vi "UPS_Monitor.vi"() -> ()   [LabVIEW 2023]
uses:
  Controls/Acquired_Datactl.ctl
  Controls/Queue_Operation_Select.ctl
  Controls/Acquired_Data.ctl
  Controls/State_and_Data.ctl
  Controls/File_Operation_Select.ctl
panel:
  out "Error_Out":errorcluster
  in  "Error_In":errorcluster
  in  "Tab Control":enum32{"PARAMETER", "DETAILS"}(tab)
  out "ACQUIRED_DATA":T1 {"Power_Consumption" scale=0.0..10.0; "Battery_Power" scale=0.0..10.0}
  out "Low_Power_Indicator":bool caption="Low Power Indicator"
  out "Waveform Graph":dbl[][](graph)
  in  "Record":bool
  in  "Stop":bool
  in  "Pause":bool
  in  "Start":bool
  # "UPS Monitor"
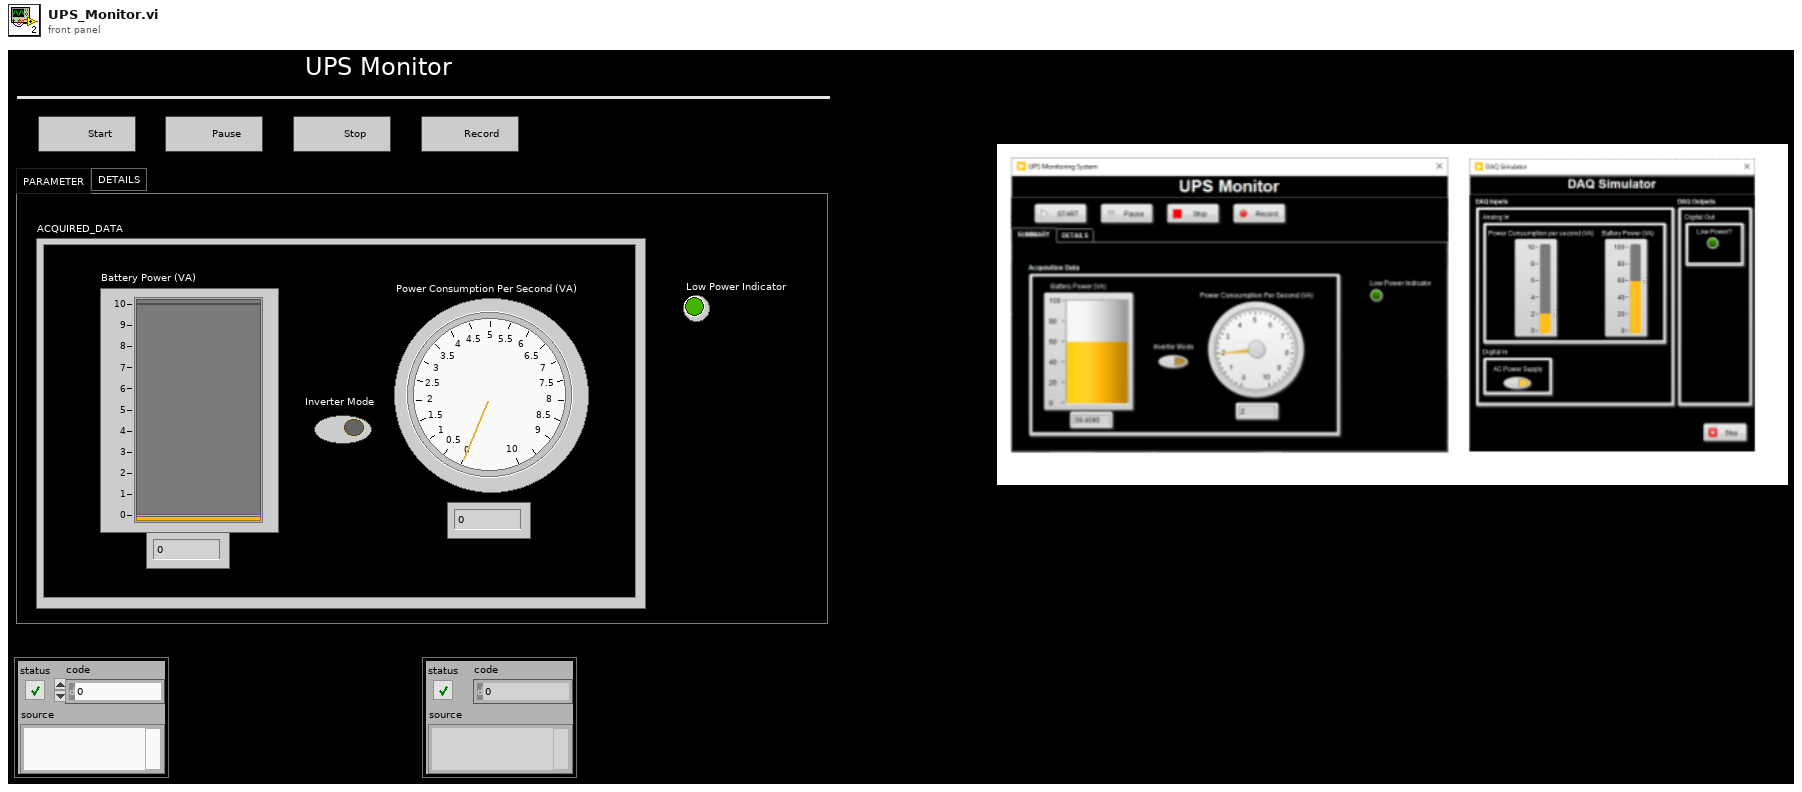
[diagram p1: front panel]
types:
  T1 = typedef "Acquired_Datactl.ctl" = cluster{"Battery_Power":dbl, "Power_Consumption":dbl, "Inverter_Mode":bool}
  T2 = typedef "Acquired_Data.ctl" = cluster{"Battery_Power":dbl, "Power_Consumption":dbl, "Inverter_Mode":bool}
  T3 = typedef "State_and_Data.ctl" = cluster{"State":string, "Data":variant}
  T4 = cluster{"ACQUIRED_DATA":T2, "Start":bool, "Pause":bool, "Record":bool, "Low_Power":bool, "Power_and_Power_Consumed":dbl[][], "State_and_Data_In":T3}
  T5 = typedef "Queue_Operation_Select.ctl" = enum16{"Obtain_Queue", "Enqueue", "Enqueue_First", "Enqueue_N", "Lossy_Enqueue", "Preview", "Queue_Status", "Dequeue", "Flush", "Release_Queue"}
  T6 = typedef "File_Operation_Select.ctl" = enum16{"Open", "Write", "Read", "Close"}
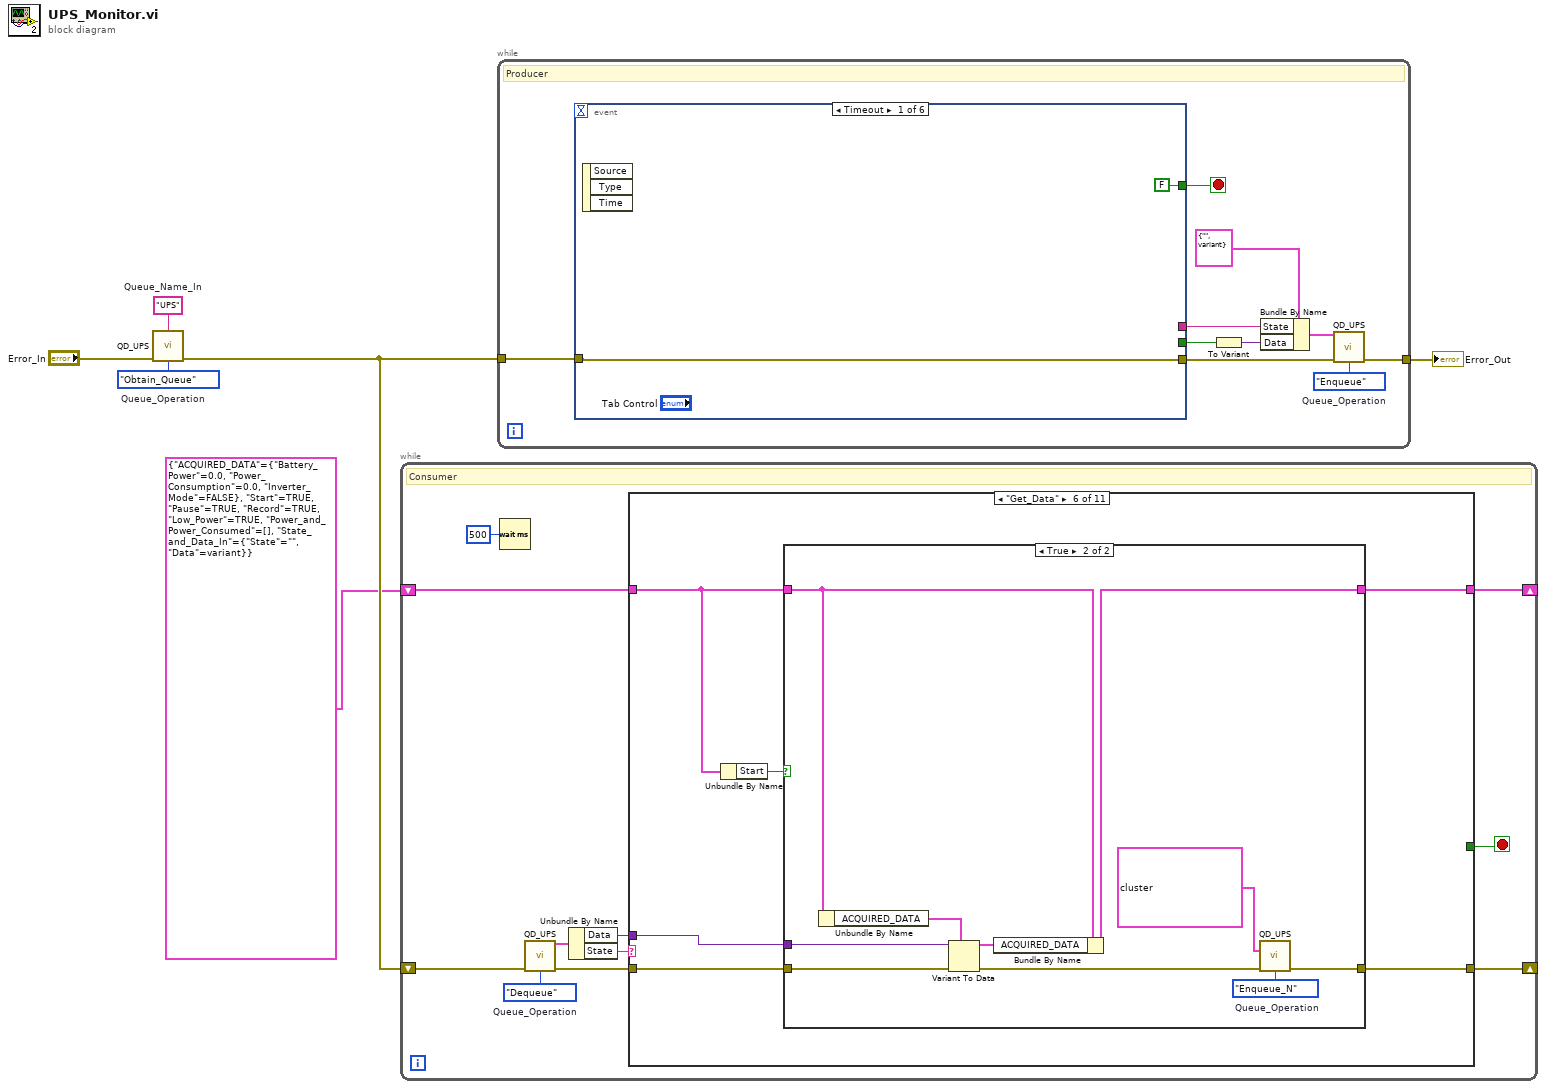
[diagram p0: block diagram]
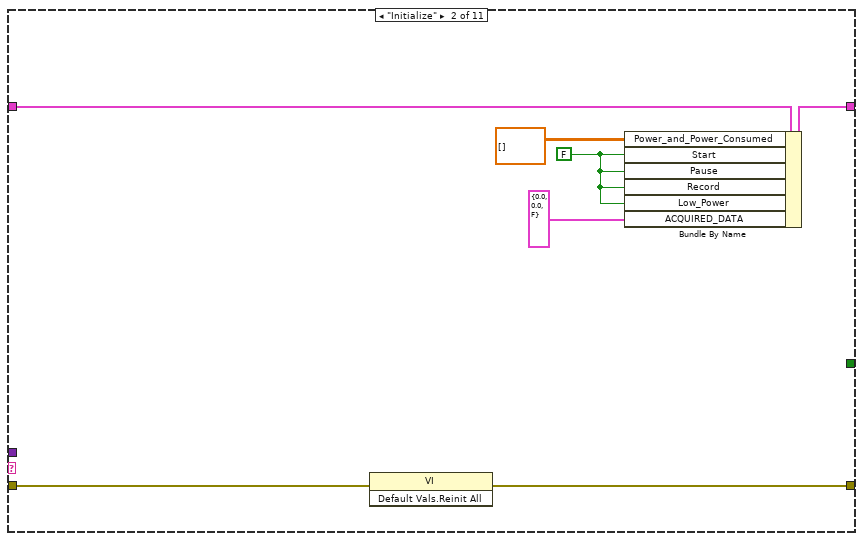
[diagram p3: hidden frame]
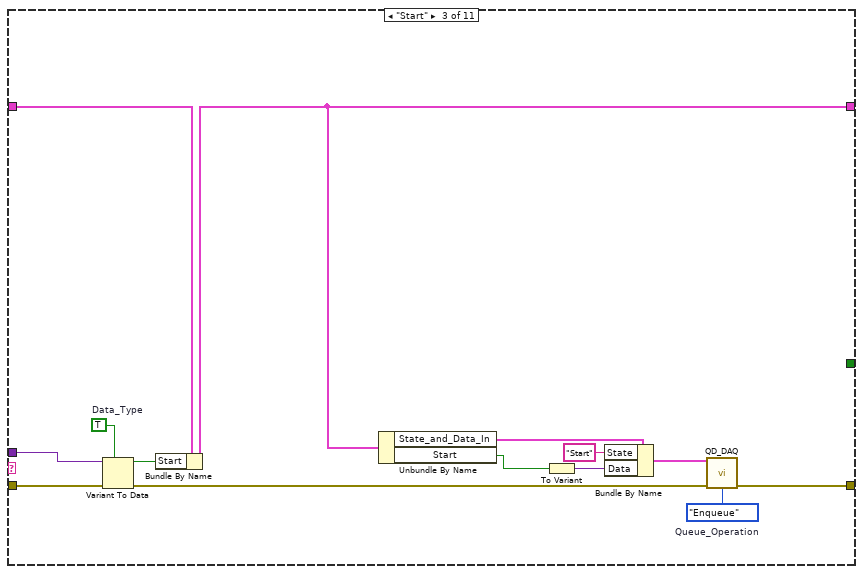
[diagram p4: hidden frame]
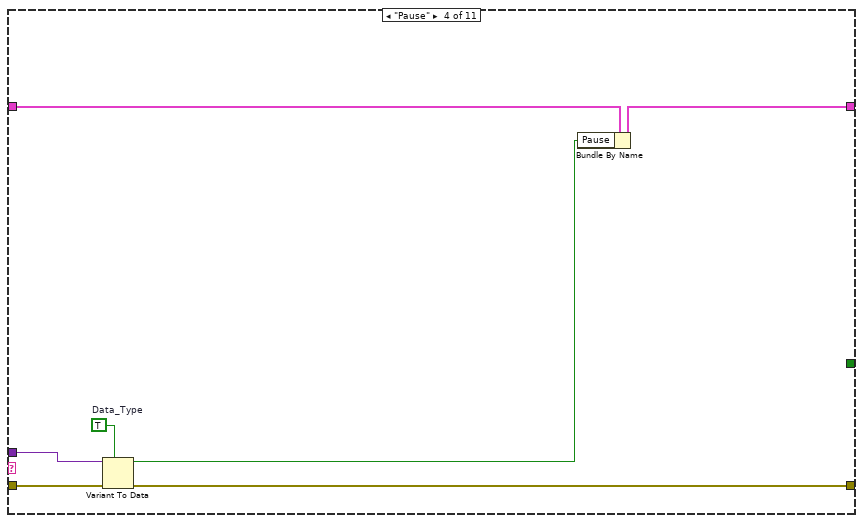
[diagram p5: hidden frame]
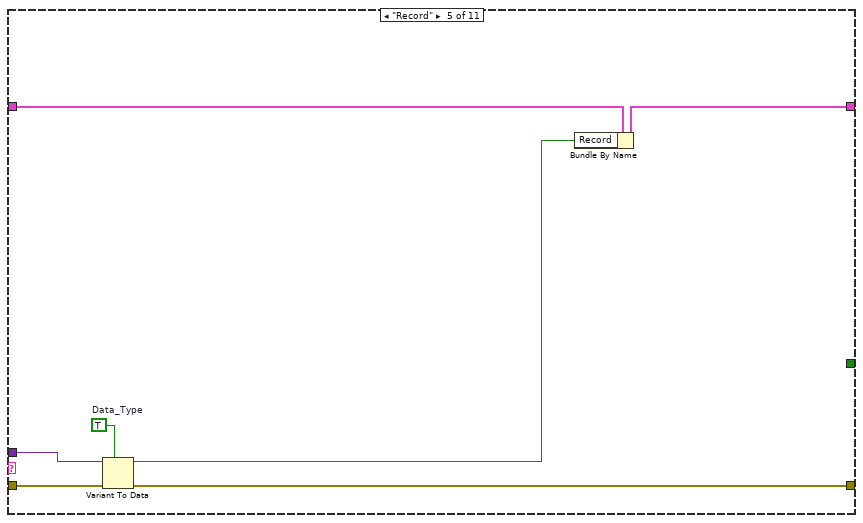
[diagram p6: hidden frame]
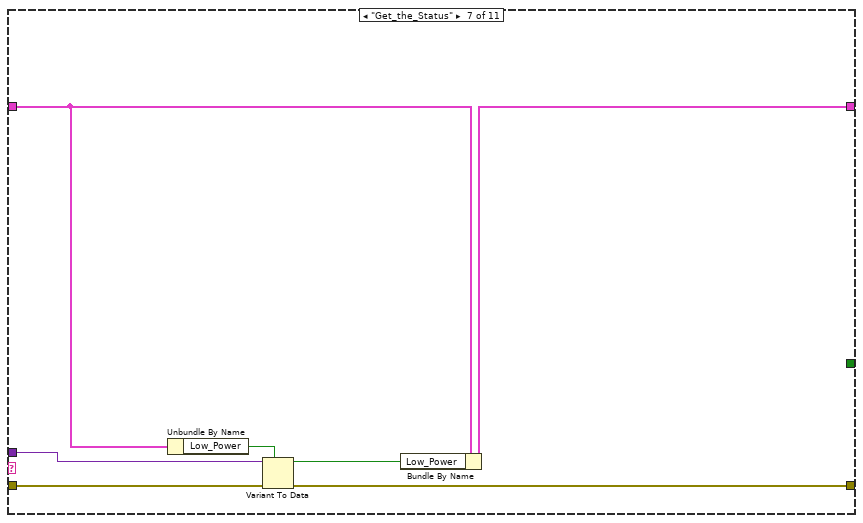
[diagram p8: hidden frame]
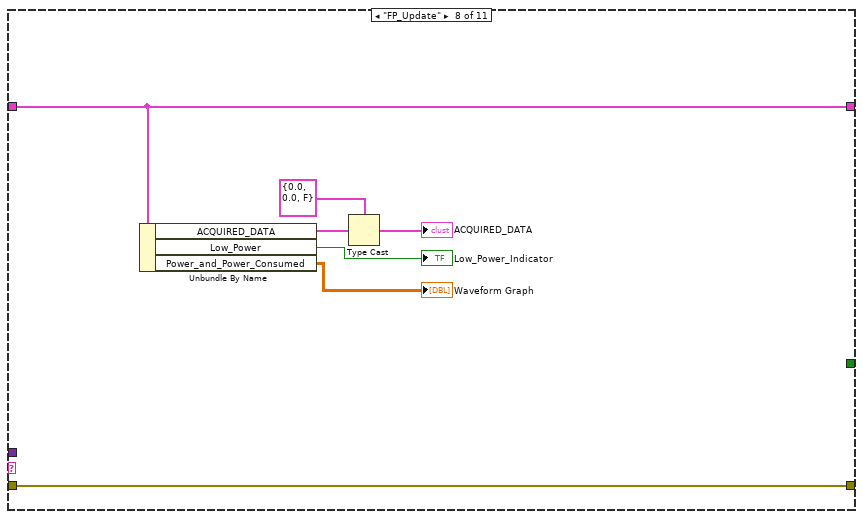
[diagram p9: hidden frame]
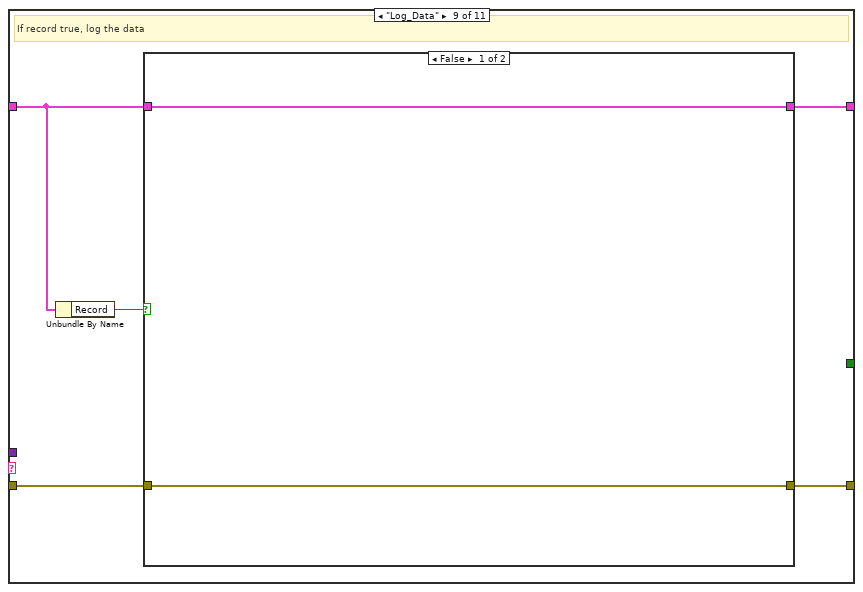
[diagram p10: hidden frame]
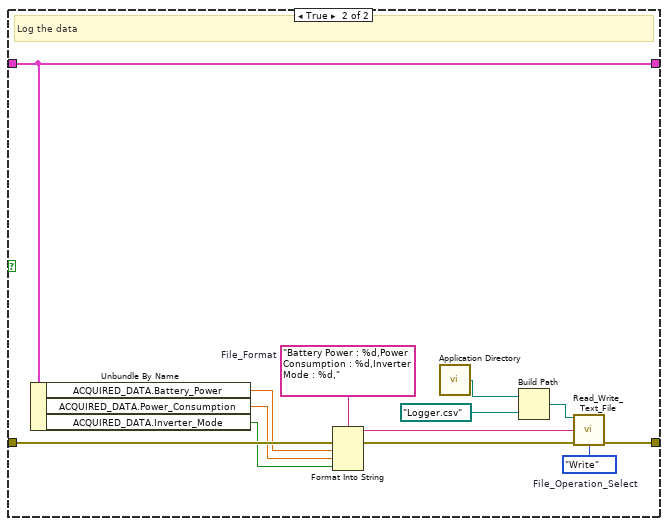
[diagram p11: hidden frame]
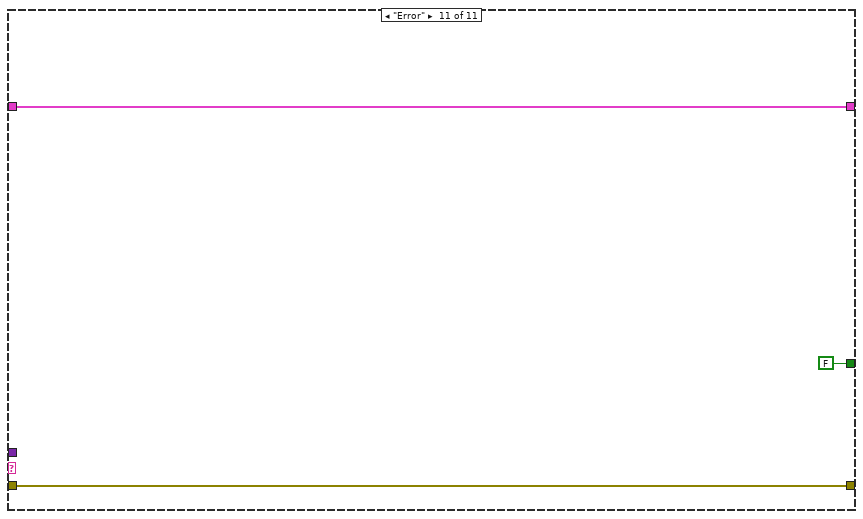
[diagram p13: hidden frame]
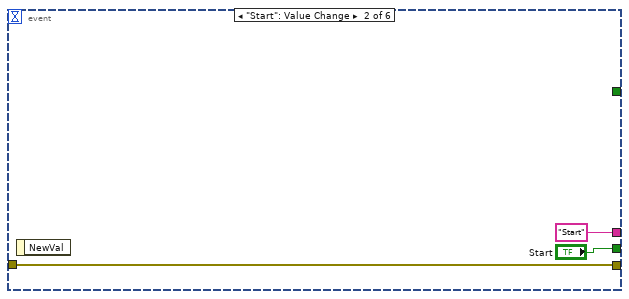
[diagram p14: hidden frame]
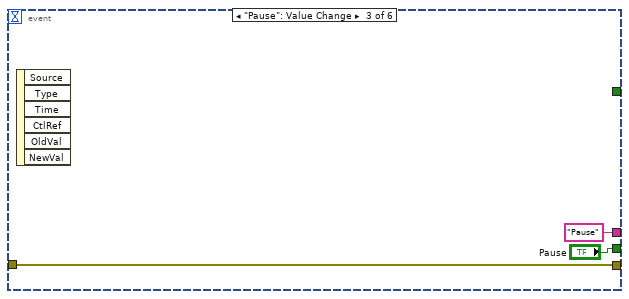
[diagram p15: hidden frame]
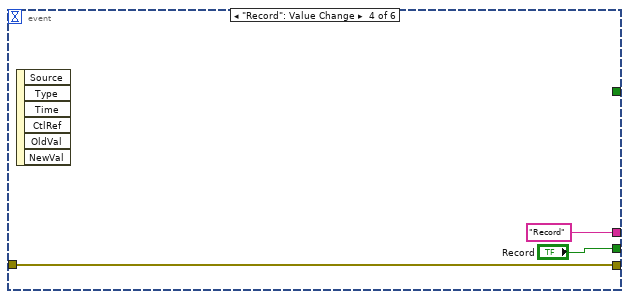
[diagram p16: hidden frame]
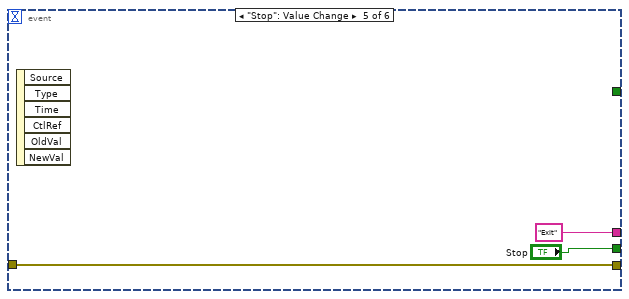
[diagram p17: hidden frame]
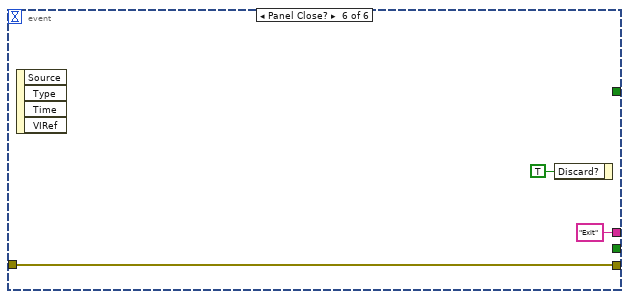
[diagram p18: hidden frame]
diagram:
  w3 = "UPS"  # Queue_Name_In
  w4 = Queue_Operation_Select."Obtain_Queue"  # Queue_Operation
  n1 = call "QD_UPS.vi"("Queue_Name_In"=w3, "Error_In"="Error_In", "Queue_Operation"=w4) -> ("Error_Out"=w2:errorcluster)  [unwired: 11 in, 1 out]
  n2 = while {
    shift-right: [w13] -> _
    shift-left: T4 {"ACQUIRED_DATA"={"Battery_Power"=0.0, "Power_Consumption"=0.0, "Inverter_Mode"=FALSE}, "Start"=TRUE, "Pause"=TRUE, "Record"=TRUE, "Low_Power"=TRUE, "Power_and_Power_Consumed"=[], "State_and_Data_In"={"State"="", "Data"=variant}} -> [w12]
    shift-right: [w8] -> _
    shift-left: w2 -> [w17]
    stop <- w10 stop-if-true
    w9 = Queue_Operation_Select."Dequeue"  # Queue_Operation
    # "Consumer"
    n3 = Wait (ms)(milliseconds to wait=u32 500) -> ()  [unwired: 1 out]
    n4 = call "QD_UPS.vi"("Error_In"=w17, "Queue_Operation"=w9) -> ("State_and_Data_Out"=w15:T3, "Error_Out"=w16:errorcluster)  [unwired: 12 in]
    n5 = Unbundle By Name(w15) -> ("Data"=w11:variant, "State"=w14:string)
    n6 = case shown="\"Get_Data\"" w14 {
      tunnel: w16 -> [w18 w25 w39 w46 w53 w60 w79 w86 w91 w107 w110]
      tunnel: [w19 w24 w32 w45 w52 w57 w78 w85 w89 w108 w111] -> w13
      tunnel: w12 -> [w19 w26 w40 w47 w54 w56 w74 w85 w88 w108 w111]
      tunnel: [w18 w20 w34 w44 w51 w59 w77 w86 w90 w107 w110] -> w8
      tunnel: w11 -> [_ _ w37 w43 w50 w58 w76 _ _ _ _]
      tunnel: [_ _ _ _ _ _ _ _ _ _ FALSE] -> w10
      frame Default {
      }
      frame "Initialize" {
        w22 = FALSE ("Start")
        n7 = invoke class="VI" method="Default Vals.Reinit All"(error in=w25) -> (error out=w20:errorcluster)  [unwired: 2 in, 2 out]
        n8 = Bundle By Name(cluster=w26, "Power_and_Power_Consumed"=dbl[][] [], "Start"=w22, "Pause"=w22, "Record"=w22, "Low_Power"=w22, "ACQUIRED_DATA"=T2 {"Battery_Power"=0.0, "Power_Consumption"=0.0, "Inverter_Mode"=FALSE}) -> (w24:T4)
      }
      frame "Start" {
        w33 = Queue_Operation_Select."Enqueue"  # Queue_Operation
        w36 = TRUE  # Data_Type
        n9 = Variant To Data(error in=w39, type=w36, Variant=w37) -> (data=w35:bool, error out=w38:errorcluster)
        n10 = Bundle By Name(cluster=w40, "Start"=w35) -> (w32:T4)
        n11 = Unbundle By Name(w32) -> ("State_and_Data_In"=w31:T3, "Start"=w28:bool)
        n12 = To Variant(anything=w28) -> (Variant=w27:variant)
        n13 = Bundle By Name(cluster=w31, "State"="Start", "Data"=w27) -> (w30:T3)
        n14 = call "QD_DAQ.vi"("Data_In"=w30, "Error_In"=w38, "Queue_Operation"=w33) -> ("Error_Out"=w34:errorcluster)  [unwired: 10 in, 2 out]
      }
      frame "Pause" {
        w42 = TRUE  # Data_Type
        n15 = Variant To Data(error in=w46, type=w42, Variant=w43) -> (data=w41:bool, error out=w44:errorcluster)
        n16 = Bundle By Name(cluster=w47, "Pause"=w41) -> (w45:T4)
      }
      frame "Record" {
        w49 = TRUE  # Data_Type
        n17 = Variant To Data(error in=w53, type=w49, Variant=w50) -> (data=w48:bool, error out=w51:errorcluster)
        n18 = Bundle By Name(cluster=w54, "Record"=w48) -> (w52:T4)
      }
      frame "Get_Data" {
        n19 = Unbundle By Name(w56) -> ("Start"=w55:bool)
        n20 = case shown="True" w55 {
          tunnel: w60 -> [w61 w72]
          tunnel: [w61 w65] -> w59
          tunnel: w58 -> [_ w70]
          tunnel: w56 -> [w62 w69]
          tunnel: [w62 w67] -> w57
          frame False {
          }
          frame True {
            w64 = Queue_Operation_Select."Enqueue_N"  # Queue_Operation
            n21 = Unbundle By Name(w69) -> ("ACQUIRED_DATA"=w68:T2)
            n22 = Variant To Data(error in=w72, type=w68, Variant=w70) -> (data=w66:T2, error out=w71:errorcluster)
            n23 = Bundle By Name(cluster=w69, "ACQUIRED_DATA"=w66) -> (w67:T4)
            n24 = call "QD_UPS.vi"("State_and_Data_N_In"=T3[] [{"State"="FP_Update", "Data"=variant}, {"State"="Log_Data", "Data"=variant}], "Error_In"=w71, "Queue_Operation"=w64) -> ("Error_Out"=w65:errorcluster)  [unwired: 11 in, 1 out]
          }
        }
      }
      frame "Get_the_Status" {
        n25 = Unbundle By Name(w74) -> ("Low_Power"=w73:bool)
        n26 = Variant To Data(error in=w79, type=w73, Variant=w76) -> (data=w75:bool, error out=w77:errorcluster)
        n27 = Bundle By Name(cluster=w74, "Low_Power"=w75) -> (w78:T4)
      }
      frame "FP_Update" {
        n28 = Unbundle By Name(w85) -> ("ACQUIRED_DATA"=w84:T2, "Low_Power"=→"Low_Power_Indicator":bool, "Power_and_Power_Consumed"=→"Waveform Graph":dbl[][])
        n29 = Type Cast(type=T1 {"Battery_Power"=0.0, "Power_Consumption"=0.0, "Inverter_Mode"=FALSE} ("ACQUIRED_DATA"), x=w84) -> (*(type *) &x=→"ACQUIRED_DATA":T1)
      }
      frame "Log_Data" {
        # "If record true, log the data"
        n30 = Unbundle By Name(w88) -> ("Record"=w87:bool)
        n31 = case shown="False" w87 {
          tunnel: w88 -> [w93 w94]
          tunnel: w91 -> [w92 w104]
          tunnel: [w92 w103] -> w90
          tunnel: [w93 w94] -> w89
          frame False {
          }
          frame True {
            w98 = "Battery Power : %d,Power Consumption : %d,Inverter Mode : %d,"  # File_Format
            w102 = File_Operation_Select."Write"  # File_Operation_Select
            # "Log the data"
            n32 = Unbundle By Name(w94) -> ("ACQUIRED_DATA.Battery_Power"=w97:dbl, "ACQUIRED_DATA.Power_Consumption"=w96:dbl, "ACQUIRED_DATA.Inverter_Mode"=w95:bool)
            n33 = Format Into String(format string=w98, error in=w104, w97, w96, w95) -> (resulting string=w99:string, error out=w101:errorcluster)  [unwired: 1 in]
            n34 = call <vilib>:"Application Directory.vi"() -> ("Application Directory"=w105:path)
            n35 = Build Path(base path=w105, name or relative path=path "Logger.csv") -> (appended path=w100:path)
            n36 = call "Read_Write_Text_File.vi"("File_Path"=w100, "Data"=w99, "Error_In"=w101, "File_Operation_Select"=w102) -> ("Error_Out"=w103:errorcluster)  [unwired: 10 in, 1 out]
          }
        }
      }
      frame "Exit" {
      }
      frame "Error" {
      }
    }
  }
  n37 = while {
    tunnel: w2 -> [w121]
    tunnel: [w116] -> w5
    stop <- w112 stop-if-true
    w115 = Queue_Operation_Select."Enqueue"  # Queue_Operation
    # "Producer"
    n38 = event shown="[0] Timeout" {
      selector: _ -> [_ _ _ _ _ _]
      dyn-events: _ -> [_ _ _ _ _ _]
      timeout: _ -> [_ _ _ _ _ _]
      tunnel: w121 -> [w123 w126 w129 w132 w135 w138]
      tunnel: [w123 w126 w129 w132 w135 w138] -> w117
      tunnel: [_ "Start" "Pause" "Record" "Stop" _] -> w114
      tunnel: [_ "Start" ("State") "Pause" ("State") "Record" ("State") "Exit" ("State") "Exit" ("State")] -> w113
      tunnel: [FALSE _ _ _ _ _] -> w112
      event Timeout {
        n39 = event-data() -> ()  [unwired: 1 in, 3 out]
      }
      event "Start": Value Change {
        n40 = event-data() -> ()  [unwired: 1 in, 1 out]
      }
      event "Pause": Value Change {
        n41 = event-data() -> ()  [unwired: 1 in, 6 out]
      }
      event "Record": Value Change {
        n42 = event-data() -> ()  [unwired: 1 in, 6 out]
      }
      event "Stop": Value Change {
        n43 = event-data() -> ()  [unwired: 1 in, 6 out]
      }
      event Panel Close? {
        n44 = event-data() -> ()  [unwired: 1 in, 4 out]
        n45 = event-data("Discard?"=TRUE) -> ()  [unwired: 1 in, 1 out]
      }
    }
    n46 = To Variant(anything=w114) -> (Variant=w120:variant)
    n47 = Bundle By Name(cluster=T3 {"State"="", "Data"=variant} ("State_and_Data_In"), "State"=w113, "Data"=w120) -> (w119:T3)
    n48 = call "QD_UPS.vi"("State_and_Data_In"=w119, "Error_In"=w117, "Queue_Operation"=w115) -> ("Error_Out"=w116:errorcluster)  [unwired: 11 in, 1 out]
  }
  "Error_Out" <- w5
